vi "getStatus.vi"(0 "HGF_Rendezvous":refnum<class "HGF_Rendezvous.lvclass">, 5 "error in (no error)":errorcluster) -> (14 "dup HGF_Rendezvous":refnum<class "HGF_Rendezvous.lvclass">, 15 "name":string, 16 "size":i32, 17 "# waiting":i32, 19 "error out":errorcluster)   [LabVIEW 2014, in "HGF_BaseClasses.lvlib" / "HGF_Rendezvous.lvclass"]
doc: "Get rendezvous status."
uses:
  HGF_Rendezvous.lvclass
  HGF_Auxiliary/HGF_Auxiliary.lvlib
  HGF_Auxiliary/Severity.ctl
  HGF_Auxiliary/ErrorCode.ctl
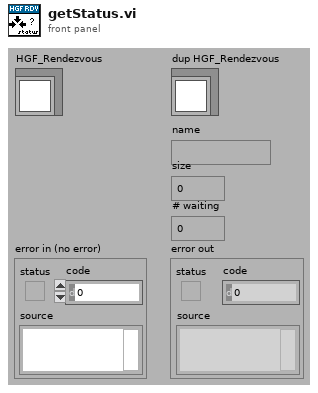
[diagram p1: front panel]
types:
  T1 = typedef "HGF_Auxiliary.lvlib/ErrorCode.ctl" = enum32{"No error", "Function not supported.", "This VI is for friends only.", "Reference object aready exisits.", "Parameter out of range.", "Not a rendezvous.", "Invalid notifier reference.", "Invalid queue reference.", "Self-Test not supported.", "Reset not supported.", "IDN query not supported.", "Error query not supported.", "Incorrect addressee.", "Object already exists.", "No class name specified", "Driver not supported", "Attribute is not writable"}
  T2 = typedef "HGF_Auxiliary.lvlib/Severity.ctl" = enum16{"Info", "Warning", "Fault", "Error", "Fatal"}
  T3 = typedef "Rendezvous RefNum" = refnum<k1>
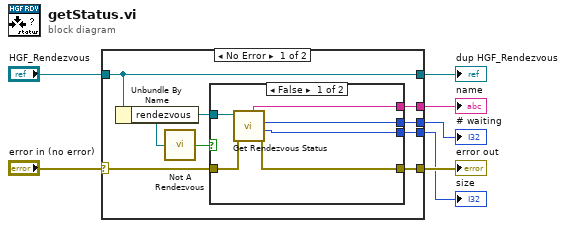
[diagram p0: block diagram]
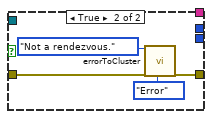
[diagram p2: hidden frame]
diagram:
  n1 = case shown="No Error" "error in (no error)" {
    selector: "error in (no error)" -> [w12 w27]
    tunnel: [w11 w27] -> w6
    tunnel: [w15 w26] -> w4
    tunnel: "HGF_Rendezvous" -> [w15 w26]
    tunnel: [w10 _] -> w3
    tunnel: [w9 _] -> w2
    tunnel: [w8 _] -> w1
    frame No Error {
      n2 = Unbundle By Name(w15) -> ("rendezvous"=w13:T3)
      n3 = call <vilib>:"Not A Rendezvous.vi"("rendezvous"=w13) -> ("not a rendezvous"=w14:bool)
      n4 = case shown="False" w14 {
        tunnel: w13 -> [w21 _]
        tunnel: w12 -> [w20 w25]
        tunnel: [w19 _] -> w9
        tunnel: [w17 w22] -> w11
        tunnel: [w18 _] -> w10
        tunnel: [w16 _] -> w8
        frame False {
          n5 = call <vilib>:"Get Rendezvous Status.vi"("error in (no error)"=w20, "rendezvous"=w21) -> ("error out"=w17:errorcluster, "size"=w16:i32, "# waiting"=w18:i32, "name"=w19:string)  [unwired: 6 out]
        }
        frame True {
          n6 = call "errorToCluster.vi"("error code"=ErrorCode."Not a rendezvous.", "error in (no error)"=w25, "severity (Error)"=Severity."Error") -> ("error out"=w22:errorcluster)  [unwired: 2 in, 14 out]
        }
      }
    }
    frame Error {
    }
  }
  "error out" <- w6
  "dup HGF_Rendezvous" <- w4
  "# waiting" <- w3
  "size" <- w1
  "name" <- w2
